vi "TTA_EXA_PeakSearch.vi"(0 "VISA resource In":refnum<visa-resource-name>, 5 "Marker\nNumber":i32, 11 "error in":errorcluster) -> (4 "VISA resource Out":refnum<visa-resource-name>, 6 "Frequency (Hz)":dbl, 8 "Amplitude (dBm)":dbl, 15 "error out":errorcluster)   [LabVIEW 2016]
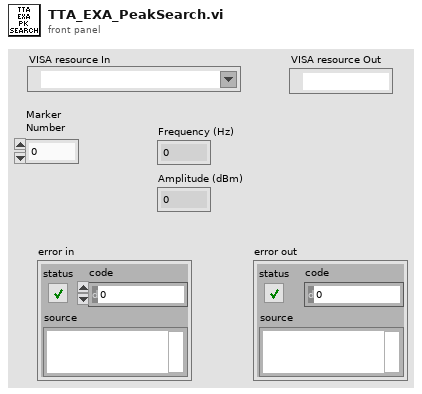
[diagram p1: front panel]
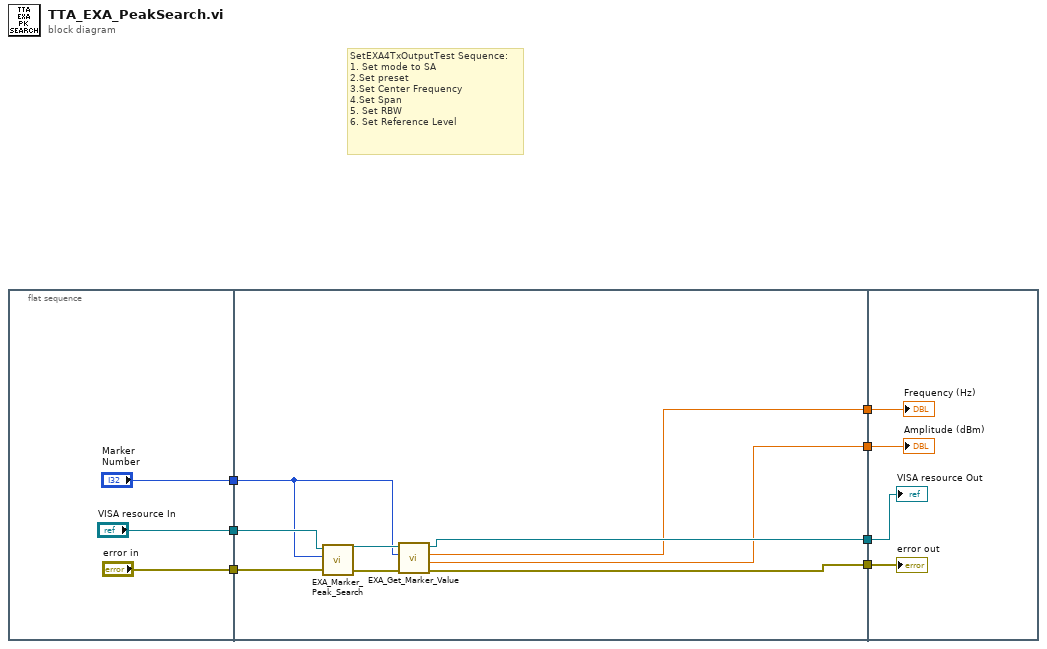
[diagram p0: block diagram]
diagram:
  # "SetEXA4TxOutputTest Sequence:\n1. Set mode to SA\n2.Set preset\n3.Set Center Frequency\n4.Set Span\n5. Set RBW\n6. Set Reference Level"
  n1 = flat-sequence {
    tunnel: ["error in"] -> w7
    tunnel: ["VISA resource In"] -> w6
    tunnel: ["Marker\nNumber"] -> w3
    tunnel: w7 -> [w19]
    tunnel: w6 -> [w18]
    tunnel: [w14] -> w5
    tunnel: [w11] -> w4
    tunnel: w3 -> [w16]
    tunnel: [w13] -> w2
    tunnel: [w12] -> w1
    tunnel: w5 -> [w23]
    tunnel: w4 -> [w22]
    tunnel: w2 -> [w21]
    tunnel: w1 -> [w20]
    frame #0 {
    }
    frame #1 {
      n2 = call "EXA_Marker_Peak_Search.vi"("error in"=w19, "Marker\nNumber"=w16, "VISA resource name"=w18) -> ("error out"=w15:errorcluster, "VISA resource name"=w17:refnum<visa-resource-name>)  [unwired: 7 in]
      n3 = call "EXA_Get_Marker_Value.vi"("error in"=w15, "Marker\nNumber"=w16, "VISA resource name"=w17) -> ("error out"=w11:errorcluster, "Amplitude (dBm)"=w12:dbl, "Frequency (Hz)"=w13:dbl, "VISA resource name"=w14:refnum<visa-resource-name>)  [unwired: 5 in]
    }
    frame #2 {
      "VISA resource Out" <- w23
      "error out" <- w22
      "Frequency (Hz)" <- w21
      "Amplitude (dBm)" <- w20
    }
  }
